vi "S8300E_BP_SlotNumber_WIH.vi"() -> ()   [LabVIEW 2011]
panel:
  out "log2":string
  out "log1":string
  out "FinalLog1":string
  out "Finalog2":string
  out "Test CMD":T1(array[cluster])
  out "Init CMD":T2(array[cluster])
  out "VISA Handle Array":refnum<visa-resource-name>[](array[refnum])
  out "VISA6":refnum<visa-resource-name>
  out "VISA9":refnum<visa-resource-name>
  out "BEGIN TIME":u32
  out "進行狀況":string
  # "S8300E BackPlane  SlotNumber"
  # "2015-5-28"
  # "Error Code:BP-SLOT"
  # "PC Com9  Baud  115200 -->S8300E MB\nPC COM6 Baud  115200 -->Test Board UART"
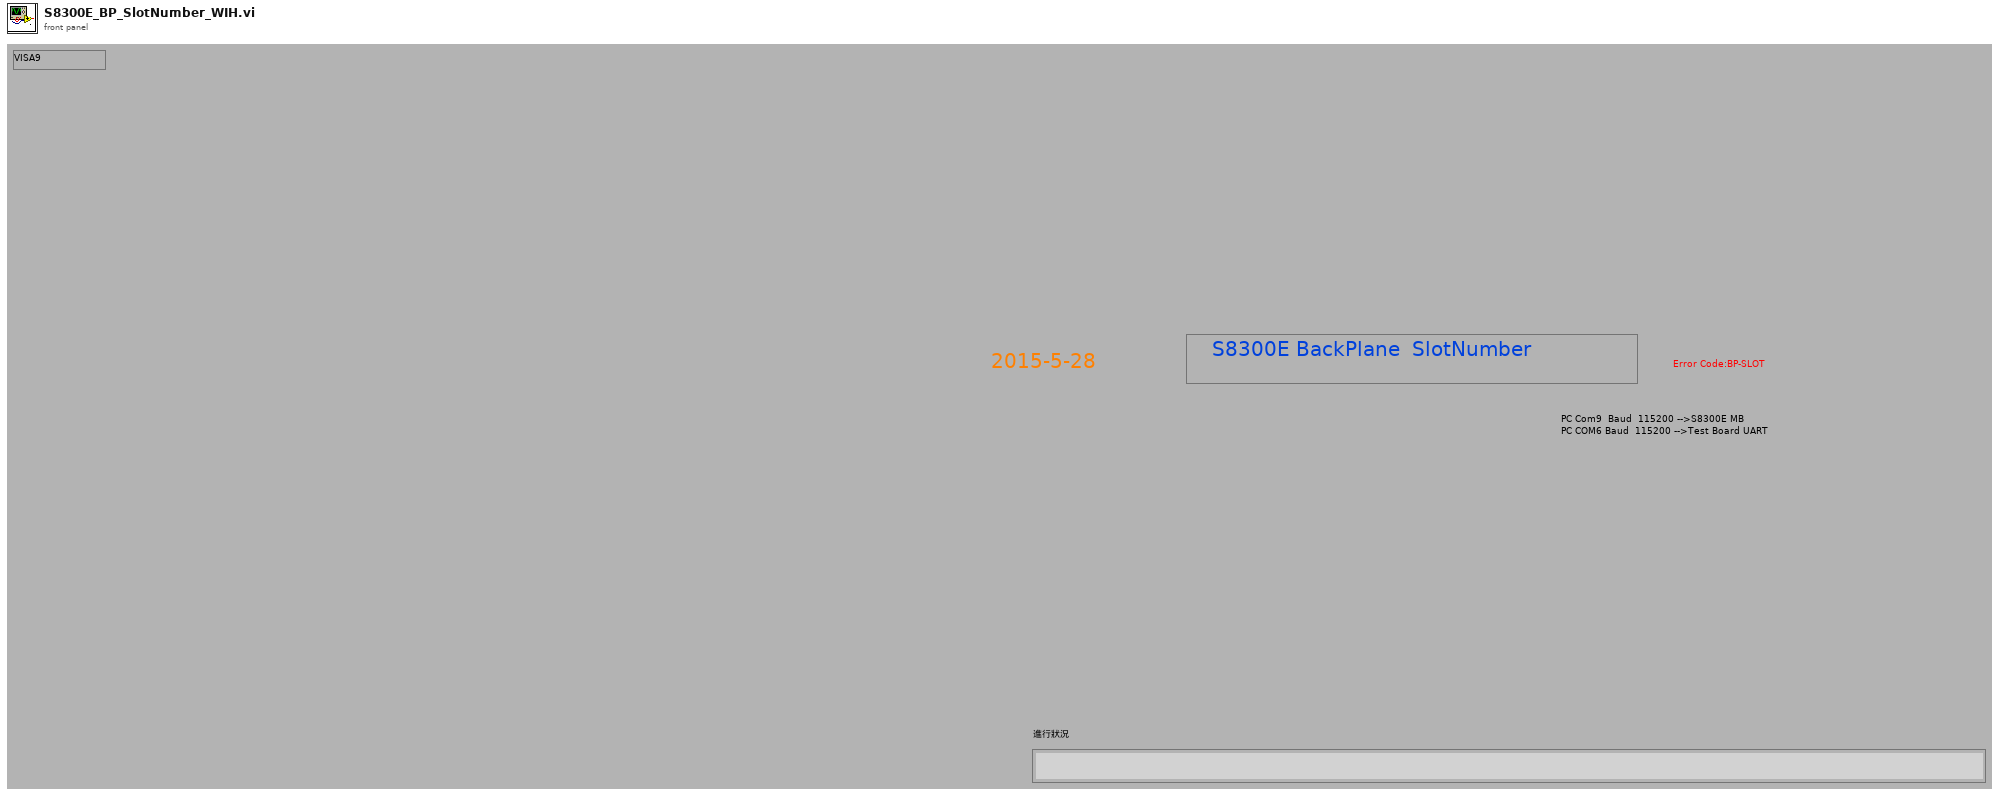
[diagram p1: front panel]
types:
  T1 = cluster{"VISA9":refnum<visa-resource-name>, "Find this String":string, "Find this String":string, "Find this String":string}[]
  T2 = cluster{"Find this String":string, "Find this String":string, "Find this String":string}[]
  T3 = cluster{string, "Find this String":string, "Find this String":string}
  T4 = cluster{"VISA6":refnum<visa-resource-name>, string, "Find this String":string, "Find this String":string}
  T5 = cluster{"VISA9":refnum<visa-resource-name>, string, "Find this String":string, "Find this String":string}
  T6 = cluster{string, "Find this String":string, "Find this String":string}[]
  T7 = cluster{"VISA9":refnum<visa-resource-name>, string, "Find this String":string, "Find this String":string}[]
  T8 = cluster{"Find this String":string, "Find this String":string, "Find this String":string}
  T9 = cluster{"VISA9":refnum<visa-resource-name>, "Find this String":string, "Find this String":string, "Find this String":string}
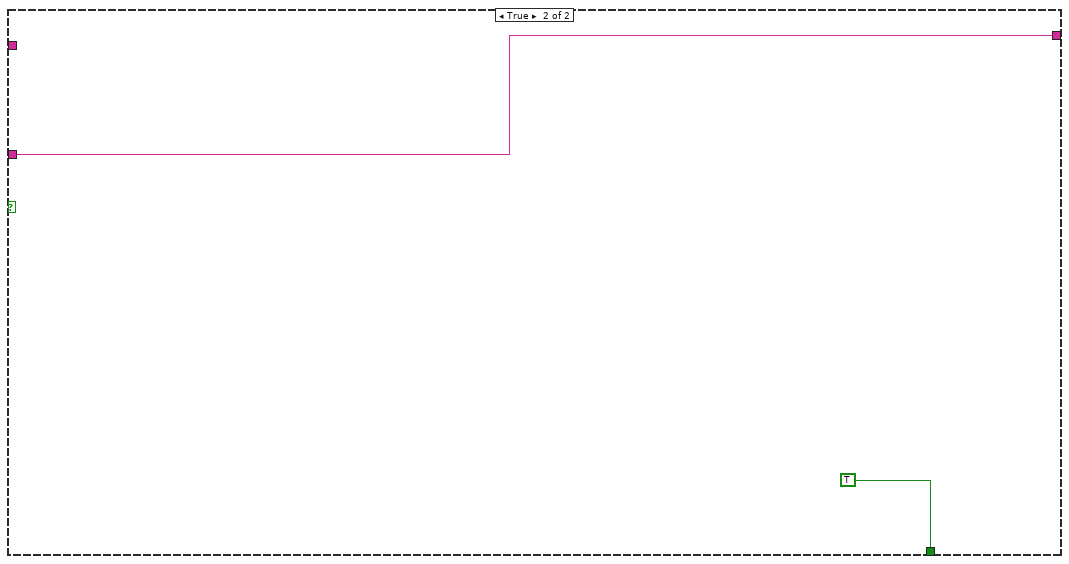
[diagram p4: hidden frame]
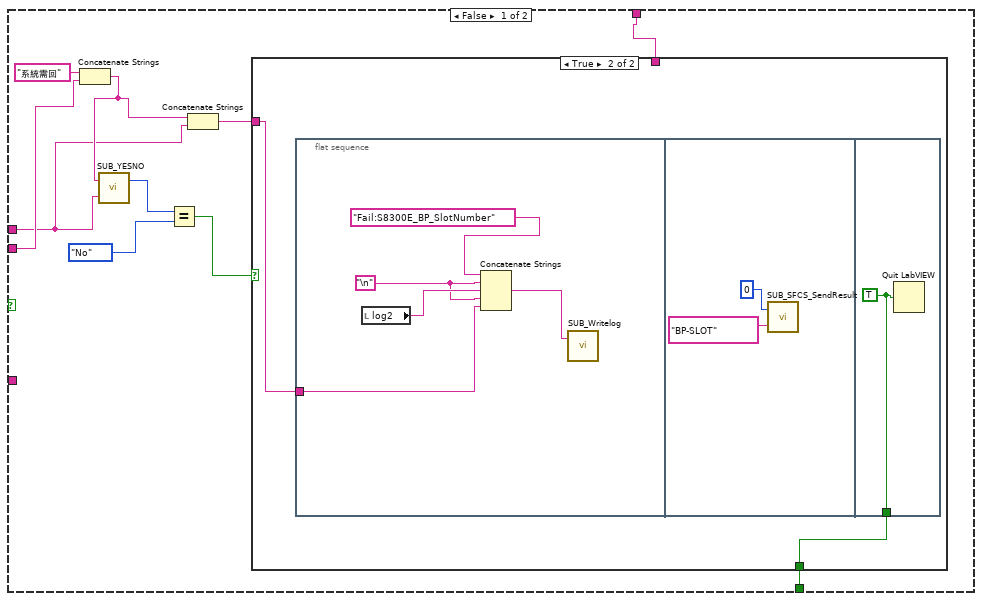
[diagram p5: hidden frame]
diagram:
  n1 = flat-sequence {
    tunnel: [w13] -> w2
    tunnel: w2 -> [w16]
    tunnel: [w93] -> w1
    tunnel: w1 -> [w94]
    frame #0 {
      n2 = Tick Count (ms)() -> (millisecond timer value=→"BEGIN TIME":u32)
    }
    frame #1 {
      n3 = Request Deallocation(TRUE ("flag")) -> ()
      n4 = property on="進行狀況" class="Str"("Blinking"=TRUE) -> ()  [unwired: 2 in, 2 out]
      "進行狀況" <- "進入測試準備中...." ("進行狀況")
    }
    frame #2 {
      n5 = call "SUB_SearchFile_inFolder.vi"("Search Filename in Folder"="S8300E_sfcs_misc.txt") -> ("File Existing True/Flase"=w7:bool)  [unwired: 1 in]
      n6 = case shown="False" w7 {
        frame False {
          n7 = flat-sequence {
            frame #0 {
              n8 = call "Display Message to User"() -> ()  [unwired: 10 in, 2 out]
            }
            frame #1 {
              n9 = call "SUB_Writelog.vi"("Pass/Fail"="Fail:S8300E_BP_SlotNumber") -> ()  [unwired: 2 in]
            }
            frame #2 {
              n10 = Quit LabVIEW(quit? (T)=TRUE) -> ()
            }
          }
        }
        frame True {
        }
      }
    }
    frame #3 {
      n11 = call "SUB_COM1_CLOSE.vi"("VISA resource name"=refnum<visa-resource-name> "COM6") -> ()  [unwired: 3 in]
    }
    frame #4 {
      n12 = call "SUB_COM1_CLOSE.vi"("VISA resource name"=refnum<visa-resource-name> "COM9") -> ()  [unwired: 3 in]
    }
    frame #5 {
      n13 = call "SUB_COM_INIT.vi"("baud rate (9600)"=u32 115200, "VISA resource name"=refnum<visa-resource-name> "COM6") -> ("VISA resource name out"=w13:refnum<visa-resource-name>)  [unwired: 1 out]
      "VISA6" <- w13
    }
    frame #6 {
      n14 = call "SUB_COM9_INIT.vi"("baud rate"=u32 115200) -> ("VISA resource name out"=w18:refnum<visa-resource-name>)  [unwired: 1 in, 1 out]
      "VISA9" <- w18
      n15 = Build Array(w16, w18) -> (→"VISA Handle Array":refnum<visa-resource-name>[])
    }
    frame #7 {
      n16 = Concatenate Strings("PT1" ("Find this String"), "\r") -> (w23:string)
      n17 = Concatenate Strings("PT2" ("Find this String"), "\r") -> (w20:string)
      n18 = local read "VISA9"() -> (w35:refnum<visa-resource-name>)
      n19 = local read "VISA6"() -> (w36:refnum<visa-resource-name>)
      n20 = Concatenate Strings("PT1" ("Find this String"), "\r") -> (w26:string)
      n21 = Concatenate Strings("./bac.sh -s", "\r") -> (w49:string)
      n22 = Concatenate Strings("./bac.sh -s", "\r") -> (w42:string)
      n23 = Bundle(w26, "Find this String"="PT1: Pass", "Find this String"="Checking COM6 Function...") -> (w39:T3)  [unwired: 1 in]
      n24 = Bundle("\r", "Find this String"="s8300e_func_test", "Find this String"="Checking COM9 Function") -> (w38:T3)  [unwired: 1 in]
      n25 = Bundle("VISA6"=w36, w23, "Find this String"="PT1: Pass", "Find this String"="G450 Output Signal Pattern1") -> (w34:T4)  [unwired: 1 in]
      n26 = Bundle("VISA9"=w35, w49, "Find this String"="PASSED=0x0A", "Find this String"="Check G450 Pattern 1") -> (w33:T5)  [unwired: 1 in]
      n27 = Bundle("VISA6"=w36, w20, "Find this String"="PT2: Pass", "Find this String"="G450 Output Signal Pattern2") -> (w32:T4)  [unwired: 1 in]
      n28 = Bundle("VISA9"=w35, w42, "Find this String"="PASSED=0x05", "Find this String"="Check G450 Pattern 2") -> (w31:T5)  [unwired: 1 in]
      n29 = Build Array(w39, w38) -> (→"Init CMD":T6)
      n30 = Build Array(w34, w33, w32, w31) -> (→"Test CMD":T7)
    }
    frame #8 {
      n31 = while {
        shift-right: [w65] -> _
        shift-left: "" -> [w66]
        i -> [w70]
        stop <- w71 stop-if-true
        w64 = "Fail" ("Find this String")
        n32 = local read "VISA6"() -> (w59:refnum<visa-resource-name>)
        n33 = Greater Or Equal?(x=w70, y=3) -> (x >= y?=w68:bool)
        n34 = Tick Count (ms)() -> (millisecond timer value=w61:u32)
        n35 = call "SUB_WR_COM1_CbyCFindString_timeout.vi"("Begin time"=w61, "Find this String"=w64, "Timeout Seccond"=3.0, "cmd string"="\r", "duplicate VISA resource name 2"=w59) -> ("Output String"=w67:string, "Found String"=w63:bool)  [unwired: 2 out]
        n36 = Concatenate Strings(w66, w67) -> (w65:string)
        n37 = call "SUB_FindSpecificString.vi"("Find this String"=w64, "String data"=w65) -> ("Found"=w62:bool)  [unwired: 2 in, 1 out]
        n38 = Or(x=w63, y=w62) -> (x .or. y?=w60:bool)
        n39 = Or(x=w60, y=w68) -> (x .or. y?=w71:bool)
      }
    }
    frame #9 {
      n40 = local read "VISA6"() -> (w74:refnum<visa-resource-name>)
      n41 = call "SUB_COM_FLUSH_TXRX.vi"("VISA resource name"=w74) -> ()  [unwired: 2 in, 1 out]
    }
    frame #10 {
      n42 = while {
        shift-right: [w78] -> _
        shift-left: "" -> [w85]
        i -> [w80]
        stop <- w79 stop-if-true
        w77 = "PT1: Pass" ("Find this String")
        n43 = local read "VISA6"() -> (w89:refnum<visa-resource-name>)
        n44 = Greater Or Equal?(x=w80, y=3) -> (x >= y?=w83:bool)
        n45 = Concatenate Strings("PT1" ("Find this String"), "\r") -> (w90:string)
        n46 = Tick Count (ms)() -> (millisecond timer value=w88:u32)
        n47 = call "SUB_WR_COM1_CbyCFindString_timeout.vi"("Begin time"=w88, "Find this String"=w77, "Timeout Seccond"=3.0, "cmd string"=w90, "duplicate VISA resource name 2"=w89) -> ("Output String"=w86:string, "Found String"=w76:bool)  [unwired: 2 out]
        n48 = Concatenate Strings(w85, w86) -> (w78:string)
        n49 = call "SUB_FindSpecificString.vi"("Find this String"=w77, "String data"=w78) -> ("Found"=w82:bool)  [unwired: 2 in, 1 out]
        n50 = Or(x=w76, y=w82) -> (x .or. y?=w81:bool)
        n51 = Or(x=w81, y=w83) -> (x .or. y?=w79:bool)
      }
    }
    frame #11 {
      n52 = Tick Count (ms)() -> (millisecond timer value=w93:u32)
    }
    frame #12 {
      n53 = while {
        shift-right: [w105] -> _
        shift-left: "" -> [w106]
        tunnel: w94 -> [w97]
        stop <- w103 stop-if-true
        n54 = local read "VISA9"() -> (w96:refnum<visa-resource-name>)
        n55 = call "SUB_COM1Wrt.vi"("VISA resource name"=w96, "write buffer"="\r") -> ("duplicate VISA resource name"=w109:refnum<visa-resource-name>)  [unwired: 1 in, 1 out]
        n56 = Tick Count (ms)() -> (millisecond timer value=w101:u32)
        n57 = Subtract(x=w101, y=w97) -> (x-y=w100:u32)
        n58 = Greater Or Equal?(x=w100, y=u32 5000) -> (x >= y?=w98:bool)
        n59 = call "SUB_ContinueCom1Read.vi"("Numeric"=1200, "duplicate VISA resource name 2"=w109) -> ("String"=w107:string)  [unwired: 1 in, 2 out]
        n60 = Concatenate Strings(w106, w107) -> (w105:string)
        n61 = call "SUB_FindSpecificString.vi"("Find this String"="S8300E", "String data"=w105) -> ("Found"=w102:bool)  [unwired: 2 in, 1 out]
        n62 = Or(x=w102, y=w98) -> (x .or. y?=w103:bool)
      }
    }
    frame #13 {
      n63 = local read "Init CMD"() -> (w112:T2)
      n64 = Array Size(array=w112) -> (size(s)=w111:i32)
      n65 = for {
        N: w111 -> [_]
        i -> [w116]
        n66 = local read "VISA Handle Array"() -> (w119:refnum<visa-resource-name>[])
        n67 = local read "Init CMD"() -> (w117:T2)
        n68 = Index Array(array=w119, index=w116) -> (element=w118:refnum<visa-resource-name>)
        n69 = Index Array(array=w117, index=w116) -> (element=w115:T8)
        n70 = while {
          tunnel: w118 -> [w121]
          tunnel: w115 -> [w134]
          shift-right: [w128] -> w113
          shift-left: "" -> [w127]
          stop <- w135 stop-if-true
          n71 = call "SUB_COM_FLUSH_TXRX.vi"("VISA resource name"=w121) -> ("VISA resource name out"=w120:refnum<visa-resource-name>)  [unwired: 2 in]
          n72 = Unbundle(w134) -> ("Find this String"=w125:string, "Find this String"=w129:string, "Find this String"=w133:string)
          n73 = Tick Count (ms)() -> (millisecond timer value=w131:u32)
          n74 = call "SUB_WR_COM1_CbyCFindString_timeout.vi"("Begin time"=w131, "Find this String"=w129, "Timeout Seccond"=5.0, "cmd string"=w125, "duplicate VISA resource name 2"=w120) -> ("Output String"=w122:string, "Found String"=w130:bool)  [unwired: 2 out]
          n75 = local write "進行狀況"(w133) -> ()
          n76 = Concatenate Strings(w125, "\n", w122) -> (w124:string)
          n77 = case shown="False" w130 {
            tunnel: [w143 TRUE] -> w135
            tunnel: w129 -> [w141 _]
            tunnel: w124 -> [w138 w158]
            tunnel: [w136 w158] -> w126
            frame False {
              n78 = Concatenate Strings("UART無正確反應!需有 " ("Status"), w141, "  字串 " ("Status")) -> (w139:string)
              n79 = call "SUB_YESNO.vi"("Debug View"=w138, "Status"=w139) -> ("yes/no"=w146:enum32{"No Selection", "Yes", "No", "None"})  [unwired: 1 in]
              n80 = Equal?(x=w146, y=enum32{"No Selection", "Yes", "No", "None"}."No") -> (x = y?=w144:bool)
              n81 = Concatenate Strings(w139, w138) -> (w137:string)
              n82 = case shown="True" w144 {
                tunnel: [_ w149] -> w143
                tunnel: w137 -> [w147 w148]
                tunnel: [w147 w148] -> w136
                frame False {
                }
                frame True {
                  n83 = flat-sequence {
                    tunnel: w148 -> [w150]
                    tunnel: [w157] -> w149
                    frame #0 {
                      n84 = local read "log1"() -> (w152:string)
                      n85 = Concatenate Strings("Fail:S8300E_BP_SlotNumber" ("Pass/Fail"), "\n", w152, w150) -> (w151:string)
                      n86 = call "SUB_Writelog.vi"("Pass/Fail"=w151) -> ()  [unwired: 2 in]
                    }
                    frame #1 {
                      n87 = call "SUB_SFCS_SendResult.vi"("ErrorCode"="UART", "PASS_Fail (1/0)"=i8 0) -> ()  [unwired: 1 out]
                    }
                    frame #2 {
                      w157 = TRUE ("quit? (T)")
                      n88 = Quit LabVIEW(quit? (T)=w157) -> ()
                    }
                  }
                }
              }
            }
            frame True {
            }
          }
          n89 = Concatenate Strings(w127, w126) -> (w128:string)
          "log1" <- w128
        }
        "FinalLog1" <- w113
      }
    }
    frame #14 {
      n90 = local read "Test CMD"() -> (w163:T1)
      n91 = Array Size(array=w163) -> (size(s)=w162:i32)
      n92 = for {
        N: w162 -> [_]
        shift-right: [w165] -> w160
        shift-left: "" -> [w164]
        i -> [w167]
        n93 = while {
          tunnel: w167 -> [w183]
          tunnel: [w179] -> w166
          stop <- w180 stop-if-true
          n94 = local read "Test CMD"() -> (w184:T1)
          n95 = Tick Count (ms)() -> (millisecond timer value=w178:u32)
          n96 = Index Array(array=w184, index=w183) -> (element=w182:T9)
          n97 = Wait (ms)(milliseconds to wait=u32 100) -> ()  [unwired: 1 out]
          n98 = Unbundle(w182) -> ("VISA9"=w169:refnum<visa-resource-name>, "Find this String"=w173:string, "Find this String"=w176:string, "Find this String"=w181:string)
          n99 = call "SUB_COM_FLUSH_TXRX.vi"("VISA resource name"=w169) -> ("VISA resource name out"=w168:refnum<visa-resource-name>)  [unwired: 2 in]
          n100 = call "SUB_WR_COM1_CbyCFindString_timeout.vi"("Begin time"=w178, "Find this String"=w176, "Timeout Seccond"=5.0, "cmd string"=w173, "duplicate VISA resource name 2"=w168) -> ("Output String"=w172:string, "Found String"=w175:bool)  [unwired: 2 out]
          n101 = local write "進行狀況"(w181) -> ()
          n102 = Concatenate Strings(w173, "\r", w172) -> (w171:string)
          n103 = case shown="True" w175 {
            tunnel: w176 -> [w190 _]
            tunnel: [w189 TRUE] -> w180
            tunnel: [w185 w206] -> w179
            tunnel: w172 -> [w187 _]
            tunnel: w171 -> [_ w206]
            frame False {
              n104 = Concatenate Strings("系統需回" ("string"), w190) -> (w188:string)
              n105 = call "SUB_YESNO.vi"("Debug View"=w187, "Status"=w188) -> ("yes/no"=w194:enum32{"No Selection", "Yes", "No", "None"})  [unwired: 1 in]
              n106 = Equal?(x=w194, y=enum32{"No Selection", "Yes", "No", "None"}."No") -> (x = y?=w192:bool)
              n107 = Concatenate Strings(w188, w187) -> (w186:string)
              n108 = case shown="True" w192 {
                tunnel: [_ w197] -> w189
                tunnel: w186 -> [w195 w196]
                tunnel: [w195 _] -> w185
                frame False {
                }
                frame True {
                  n109 = flat-sequence {
                    tunnel: w196 -> [w198]
                    tunnel: [w205] -> w197
                    frame #0 {
                      w200 = "\n"
                      n110 = local read "log2"() -> (w201:string)
                      n111 = Concatenate Strings("Fail:S8300E_BP_SlotNumber" ("Pass/Fail"), w200, w201, w200, w198) -> (w199:string)
                      n112 = call "SUB_Writelog.vi"("Pass/Fail"=w199) -> ()  [unwired: 2 in]
                    }
                    frame #1 {
                      n113 = call "SUB_SFCS_SendResult.vi"("ErrorCode"="BP-SLOT", "PASS_Fail (1/0)"=i8 0) -> ()  [unwired: 1 out]
                    }
                    frame #2 {
                      w205 = TRUE ("quit? (T)")
                      n114 = Quit LabVIEW(quit? (T)=w205) -> ()
                    }
                  }
                }
              }
            }
            frame True {
            }
          }
        }
        n115 = Concatenate Strings(w164, w166) -> (w165:string)
        "log2" <- w165
      }
      "Finalog2" <- w160
    }
    frame #15 {
      n116 = call "SUB_COM1_CLOSE.vi"("VISA resource name"=refnum<visa-resource-name> "COM9") -> ()  [unwired: 3 in]
    }
    frame #16 {
      n117 = call "SUB_COM1_CLOSE.vi"("VISA resource name"=refnum<visa-resource-name> "COM6") -> ()  [unwired: 3 in]
    }
    frame #17 {
      w211 = "***Not Good ***" ("replace string (\"\")")
      w217 = "\n"
      n118 = local read "FinalLog1"() -> (w219:string)
      n119 = local read "Finalog2"() -> (w218:string)
      n120 = local read "BEGIN TIME"() -> (w222:u32)
      n121 = Tick Count (ms)() -> (millisecond timer value=w221:u32)
      n122 = call "SUB_CAL_TESTTIME.vi"("Test Item name"="S8300E_BP_SlotNumber", "Stop tick time"=w221, "Start tick time"=w222) -> ("Test Time output"=w216:string)  [unwired: 2 in]
      n123 = Concatenate Strings("Pass:S8300E_BP_SlotNumber", w217, w219, w217, w218, w217, w216) -> (w215:string)
      n124 = call "SUB_SEARCH_REPLACE_STR.vi"("replace string (\"\")"=w211, "search string"="FAILED", "input string"=w215) -> ("result string"=w213:string)  [unwired: 2 in]
      n125 = call "SUB_SEARCH_REPLACE_STR.vi"("replace string (\"\")"=w211, "search string"="FAIL", "input string"=w213) -> ("result string"=w210:string)  [unwired: 2 in]
      n126 = call "SUB_Writelog.vi"("Pass/Fail"=w210) -> ()  [unwired: 2 in]
    }
    frame #18 {
      n127 = Quit LabVIEW(quit? (T)=TRUE ("stop? (T)")) -> ()
    }
  }
